vi "test-find-path.vi"() -> ()   [LabVIEW 2019]
uses:
  <vilib>/Rock Robotics/WPI/ThirdParty/JAS_Junk/TrajLib/TypeDef/TRANSLATION2D.ctl
  <vilib>/Rock Robotics/WPI/ThirdParty/MJansen/PathPlanner/TypeDef/PathPlannerGoalEndState.ctl
  <vilib>/Rock Robotics/WPI/ThirdParty/JAS_Junk/TrajLib/TypeDef/ROTATION2D.ctl
  <vilib>/Rock Robotics/WPI/ThirdParty/MJansen/PathPlanner/TypeDef/PathPlannerPath.ctl
  <vilib>/Rock Robotics/WPI/ThirdParty/MJansen/PathPlanner/TypeDef/PathPlannerRotationTarget.ctl
  <vilib>/Rock Robotics/WPI/ThirdParty/MJansen/PathPlanner/TypeDef/PathPlannerConstraintsZone.ctl
  <vilib>/Rock Robotics/WPI/ThirdParty/MJansen/PathPlanner/TypeDef/PathPlannerPathConstraints.ctl
  <vilib>/Rock Robotics/WPI/ThirdParty/MJansen/PathPlanner/TypeDef/PathPlannerEventMarker.ctl
  <vilib>/Rock Robotics/WPI/ThirdParty/MJansen/PathPlanner/TypeDef/PathPlannerCommandUtil.ctl
  <vilib>/Rock Robotics/WPI/ThirdParty/MJansen/PathPlanner/ENum/PathPlanner_CommandUtilType_ENUM.ctl
  <vilib>/Rock Robotics/WPI/ThirdParty/MJansen/PathPlanner/TypeDef/PathPlannerPathPoint.ctl
  <vilib>/Rock Robotics/WPI/ThirdParty/JAS_Junk/TrajLib/TypeDef/CHASSIS_SPEEDS.ctl
  <vilib>/Rock Robotics/WPI/ThirdParty/MJansen/PathPlanner/VI/PathPlanner_GridPosition_Get.vi
  <vilib>/Rock Robotics/WPI/ThirdParty/JAS_Junk/TrajLib/Translation2d_Create.vi
  <vilib>/Rock Robotics/WPI/ThirdParty/MJansen/PathPlanner/VI/PathPlanner_PathFinder_Globals.vi
  <vilib>/robotics/Navigation/shared/WorldMap/OccupancyGridWorldMap/NI_Robotics_OccupancyGridWorldMap.lvclass
  <vilib>/robotics/Navigation/shared/MapNode/AbstractDstarNode/NI_Robotics_AbstractDstarNode.lvclass
  <vilib>/Rock Robotics/WPI/ThirdParty/MJansen/PathPlanner/PathPlanner24.lvlib
  <vilib>/Rock Robotics/WPI/ThirdParty/JAS_Junk/TrajLib/Trajectory_Library.lvlib
panel:
  out "Extract Simplified Path Size":i32
  out "Do Reset Err Count":i64
  out "Do Minor Err Count":i64
  out "Do Major Err Count":i64
  out "Extract Path Size":i32
  out "Field":cluster{dbl[], dbl[]}[](graph)=[{array[568 elements], array[568 elements]}, {[1.65, 1.9499999999999997, 2.25, 2.55, 2.8499999999999996, 3.15, 3.4499999999999997, 3.7499999999999996, 4.05, 4.3500000000000005, 4.65, 4.95, 5.25, 5.55, 5.8500000000000005, 6.15, 6.45, 6.75, 7.05, 7.35, 7.65, 7.95, 8.25, 8.55, 8.85, 9.15, 9.45, 9.75, 10.05, 10.35, 10.65, 10.95, 11.25, 11.55, 11.85, 12.15, 12.45, 12.75, 13.05, 13.35, 13.65], [1.65, 1.65, 1.65, 1.65, 1.65, 1.65, 1.65, 1.65, 1.65, 1.65, 1.65, 1.65, 1.65, 1.65, 1.65, 1.65, 1.65, 1.65, 1.65, 1.65, 1.65, 1.65, 1.65, 1.65, 1.65, 1.65, 1.65, 1.65, 1.65, 1.65, 1.65, 1.65, 1.65, 1.65, 1.65, 1.65, 1.65, 1.65, 1.65, 1.65, 1.65]}, {[1.65, 13.65], [1.65, 1.65]}, {[1.5, 2.1072631250000002, 2.7161800000000005, 3.326566875, 3.9382400000000004, 4.551015625, 5.1647099999999995, 5.779139375, 6.39412, 7.009468125, 7.624999999999998, 8.240531874999999, 8.855879999999999, 9.470860625, 10.08529, 10.698984375000002, 11.311760000000003, 11.923433125000003, 12.533820000000002, 13.142736875000004, 13.75], [1.5, 1.5, 1.5, 1.5, 1.5, 1.5, 1.5, 1.5, 1.5, 1.5, 1.5, 1.5, 1.5, 1.5, 1.5, 1.5, 1.5, 1.5, 1.5, 1.5, 1.5]}, {array[568 elements], array[568 elements]}]
  out "Error_No_Path":bool
  out "New Path Available":bool
  out "Loop Count":i32
  out "TerminateWorker":bool
  out "Do Work Count":i64
  out "Do Reset Count":i64
  out "Do Minor Count":i64
  out "Do Major Count":i64
  out "PathPlannerPath":T1={"BezierPoints"=[], "PreviewStartingRotation"={"VALUE"=0.0, "COS"=1.0, "SIN"=0.0}, "Reversed"=FALSE, "RotationTargets"=[], "ConstraintZones"=[], "EventMarkers"=[], "GlobalConstraints"={"MaxVelocityMps;"=0.0, "MaxAccelerationMpsSq;"=0.0, "MaxAngularVelRadPsEc;"=0.0, "MaxAngularAccRadPSecSq"=0.0, "Exists"=FALSE}, "GoalEndState"={"Velocity"=0.0, "Rotation"={"VALUE"=0.0, "COS"=1.0, "SIN"=0.0}}, "AllPoints"=[]} {"AllPoints"."HolonomicRotation"."SIN" format="%13.4f"; "AllPoints"."HolonomicRotation"."COS" format="%13.4f"; "AllPoints"."HolonomicRotation"."VALUE" format="%13.4f"; "AllPoints"."Position"."Y" format="%14.3f"; "AllPoints"."Position"."X" format="%14.3f"; "GoalEndState"."Rotation"."SIN" format="%13.4f"; "GoalEndState"."Rotation"."COS" format="%13.4f"; "GoalEndState"."Rotation"."VALUE" format="%13.4f"; "EventMarkers"."lastRobotPos"."Y" format="%14.3f"; "EventMarkers"."lastRobotPos"."X" format="%14.3f"; "EventMarkers"."markerPos"."Y" format="%14.3f"; "EventMarkers"."markerPos"."X" format="%14.3f"; "RotationTargets"."target"."SIN" format="%13.4f"; "RotationTargets"."target"."COS" format="%13.4f"; "RotationTargets"."target"."VALUE" format="%13.4f"; "PreviewStartingRotation"."SIN" format="%13.4f"; "PreviewStartingRotation"."COS" format="%13.4f"; "PreviewStartingRotation"."VALUE" format="%13.4f"; "BezierPoints"."Y" format="%14.3f"; "BezierPoints"."X" format="%14.3f"}
  in  "GoalEndState":T10={"Velocity"=0.0, "Rotation"={"VALUE"=0.0, "COS"=1.0, "SIN"=0.0}} {"Rotation"."SIN" format="%13.4f"; "Rotation"."COS" format="%13.4f"; "Rotation"."VALUE" format="%13.4f"}
  in  "Goal Position":T2={"X"=14.0, "Y"=7.0} {"Y" step=0.25 format="%14.3f"; "X" step=0.25 format="%14.3f"}
  in  "StartPosition":T2={"X"=1.5, "Y"=1.5} {"Y" step=0.25 format="%14.3f"; "X" step=0.25 format="%14.3f"}
  out "NewPathAvailLastCheck":i32
  out "NewPathAvailCount":i32
  out "BackGroundInitialized":bool
  out "Main Program Name":string
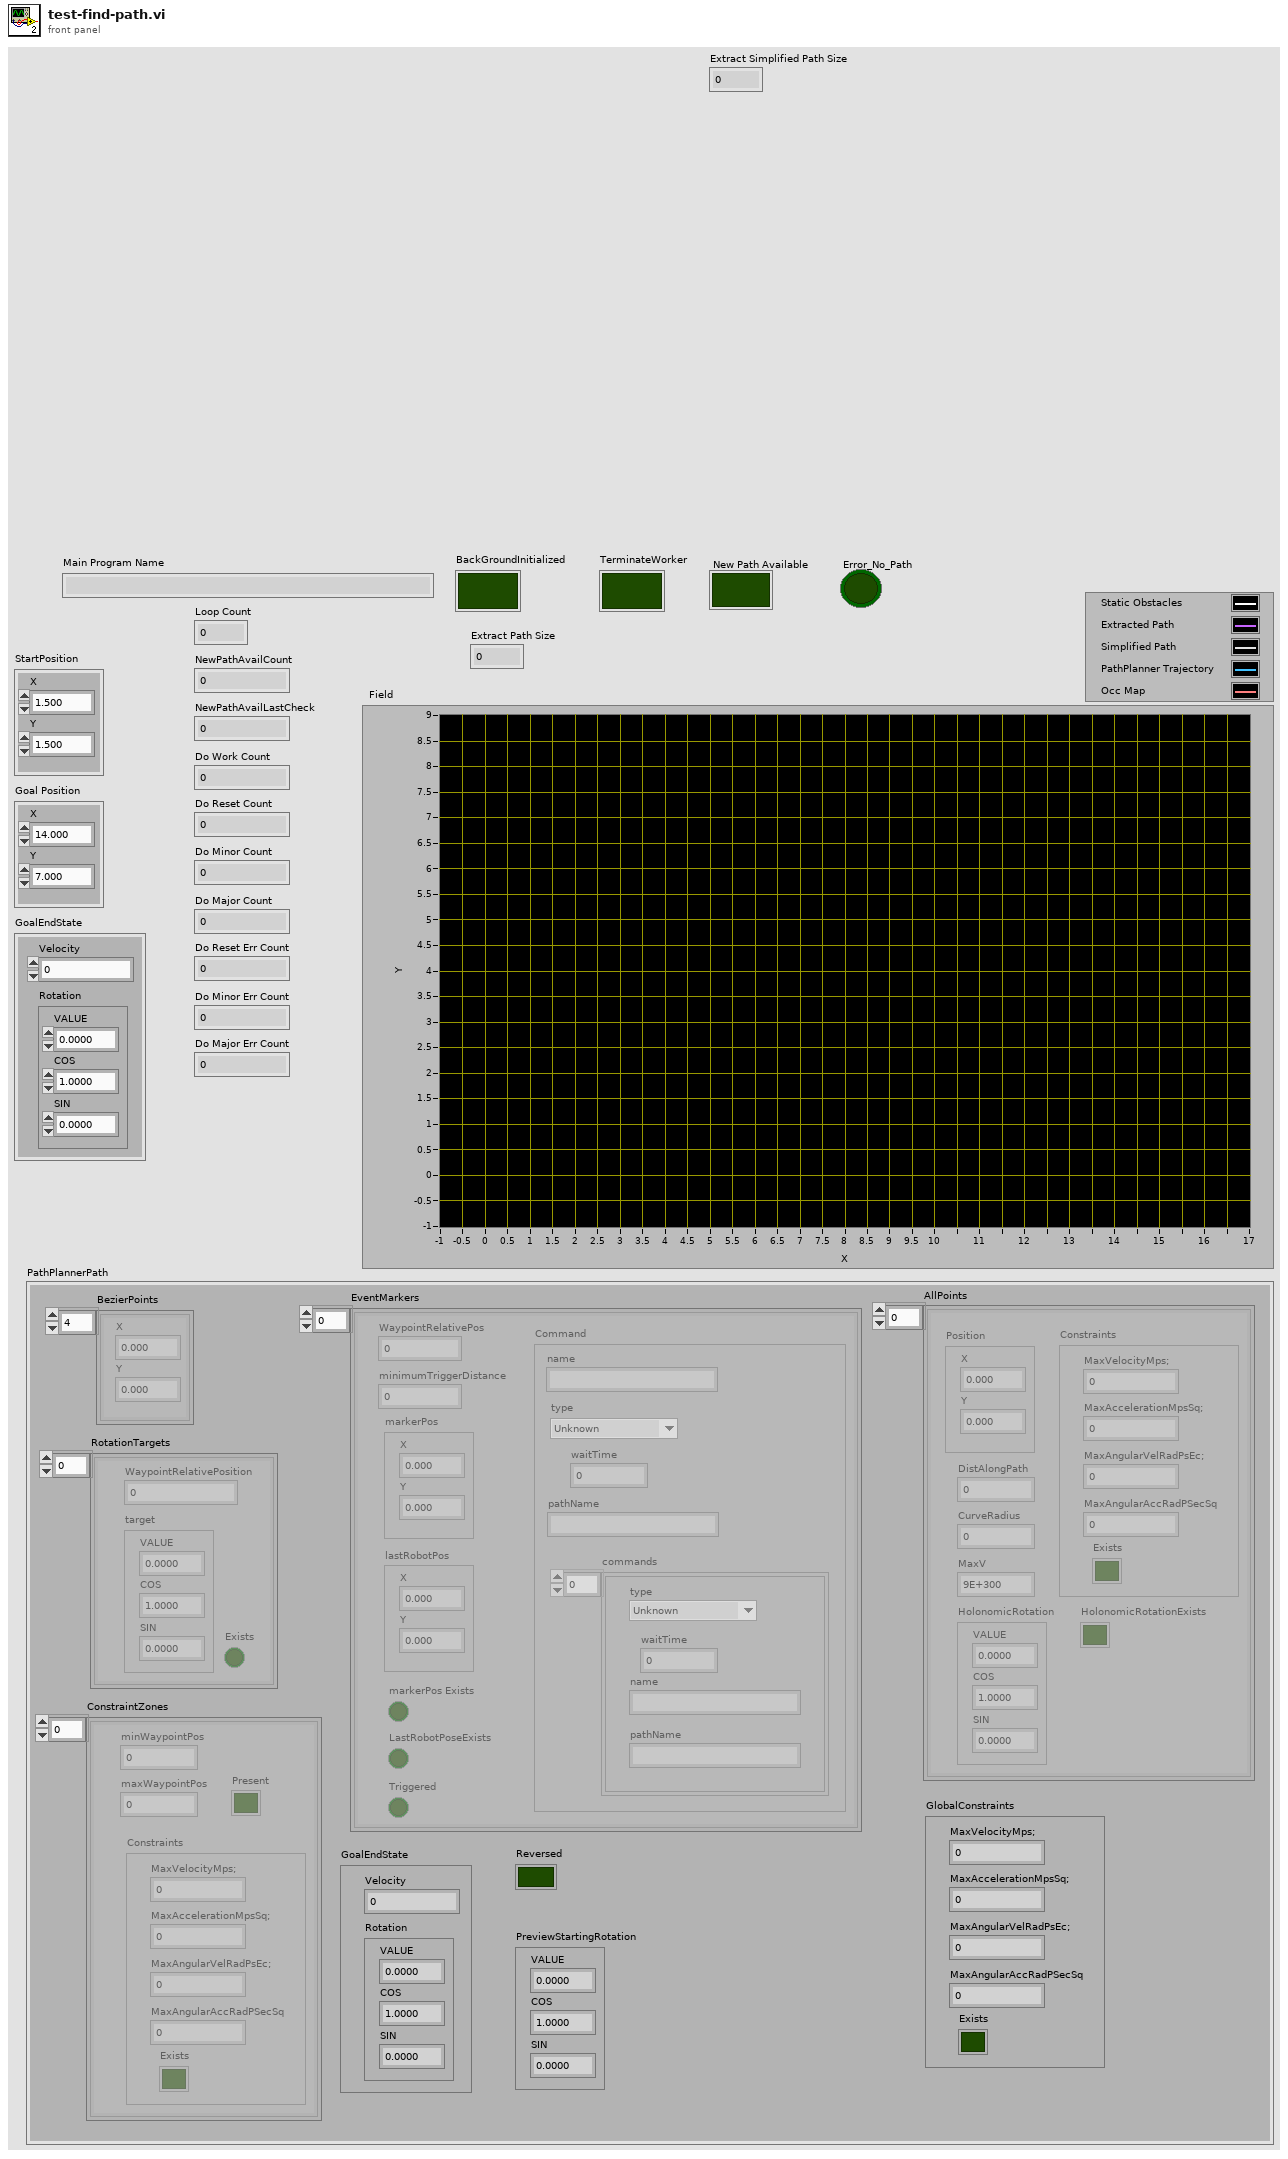
[diagram p1: front panel]
types:
  T1 = typedef "PathPlanner24.lvlib/PathPlannerPath.ctl" = cluster{"BezierPoints":T2[], "PreviewStartingRotation":T3, "Reversed":bool, "RotationTargets":T4[], "ConstraintZones":T5[], "EventMarkers":T7[], "GlobalConstraints":T6, "GoalEndState":T10, "AllPoints":T11[]}
  T2 = typedef "Trajectory_Library.lvlib/TRANSLATION2D.ctl" = cluster{"X":dbl, "Y":dbl}
  T3 = typedef "Trajectory_Library.lvlib/ROTATION2D.ctl" = cluster{"VALUE":dbl, "COS":dbl, "SIN":dbl}
  T4 = typedef "PathPlanner24.lvlib/PathPlannerRotationTarget.ctl" = cluster{"target":T3, "WaypointRelativePosition":dbl, "Exists":bool}
  T5 = typedef "PathPlanner24.lvlib/PathPlannerConstraintsZone.ctl" = cluster{"minWaypointPos":dbl, "maxWaypointPos":dbl, "Constraints":T6, "Present":bool}
  T6 = typedef "PathPlanner24.lvlib/PathPlannerPathConstraints.ctl" = cluster{"MaxVelocityMps;":dbl, "MaxAccelerationMpsSq;":dbl, "MaxAngularVelRadPsEc;":dbl, "MaxAngularAccRadPSecSq":dbl, "Exists":bool}
  T7 = typedef "PathPlanner24.lvlib/PathPlannerEventMarker.ctl" = cluster{"WaypointRelativePos":dbl, "minimumTriggerDistance":dbl, "markerPos":T2, "lastRobotPos":T2, "Command":T8, "markerPos Exists":bool, "LastRobotPoseExists":bool, "Triggered":bool}
  T8 = typedef "PathPlanner24.lvlib/PathPlannerCommandUtil.ctl" = cluster{"waitTime":dbl, "name":string, "pathName":string, "commands":cluster{"type":T9, "waitTime":dbl, "name":string, "pathName":string}[], "type":T9}
  T9 = typedef "PathPlanner24.lvlib/PathPlanner_CommandUtilType_ENUM.ctl" = enum16{"Unknown", "Wait", "Named", "Path", "Sequential", "Parallel", "Race", "Deadline"}
  T10 = typedef "PathPlanner24.lvlib/PathPlannerGoalEndState.ctl" = cluster{"Velocity":dbl, "Rotation":T3}
  T11 = typedef "PathPlanner24.lvlib/PathPlannerPathPoint.ctl" = cluster{"Position":T2, "HolonomicRotation":T3, "DistAlongPath":dbl, "CurveRadius":dbl, "MaxV":dbl, "Constraints":T6, "HolonomicRotationExists":bool}
  T12 = typedef "Trajectory_Library.lvlib/CHASSIS_SPEEDS.ctl" = cluster{"vX":dbl, "vY":dbl, "vOmega":dbl}
  T13 = cluster{"DoResetErrCount":i64, "DoResetCount":i64, "DoMinorErrCount":i64, "DoMinorCount":i64, "DoMajorErrCount":i64, "DoMajorCount":i64, "DoWorkLoopCount":i64, "BackGroundInitialized":bool, "TerminateWorker":bool}
  T14 = typedef "PathPlanner24.lvlib/PathPlannerFinderGridPosition.ctl" = cluster{"X":i32, "Y":i32}
  T15 = cluster{"ExtractedPath":T14[], "ExtractedPathSimplified":T14[], "ExtractedFieldPosPath":T2[], "CurrentPath":T2[], "Obstacles":set{T14}, "StaticOccupancyGrid":refnum<data-value>, "path references":refnum<data-value>[], "Main Program Name":string}
  T16 = typedef "PathPlanner24.lvlib/PathPlannerTrajectory.ctl" = cluster{"States":T17[]}
  T17 = typedef "PathPlanner24.lvlib/PathPlannerTrajectoryState.ctl" = cluster{"TimeSeconds":dbl, "VelocityMPS":dbl, "AccerationMpsSq":dbl, "HeadingAngularVelRadPerSec":dbl, "PositionMeters":T2, "Heading":T3, "TargetHolonomicRotation":T3, "CurvatureRadPerMeter":dbl, "PathPlannerConstraints":T6, "DeltaPos":dbl}
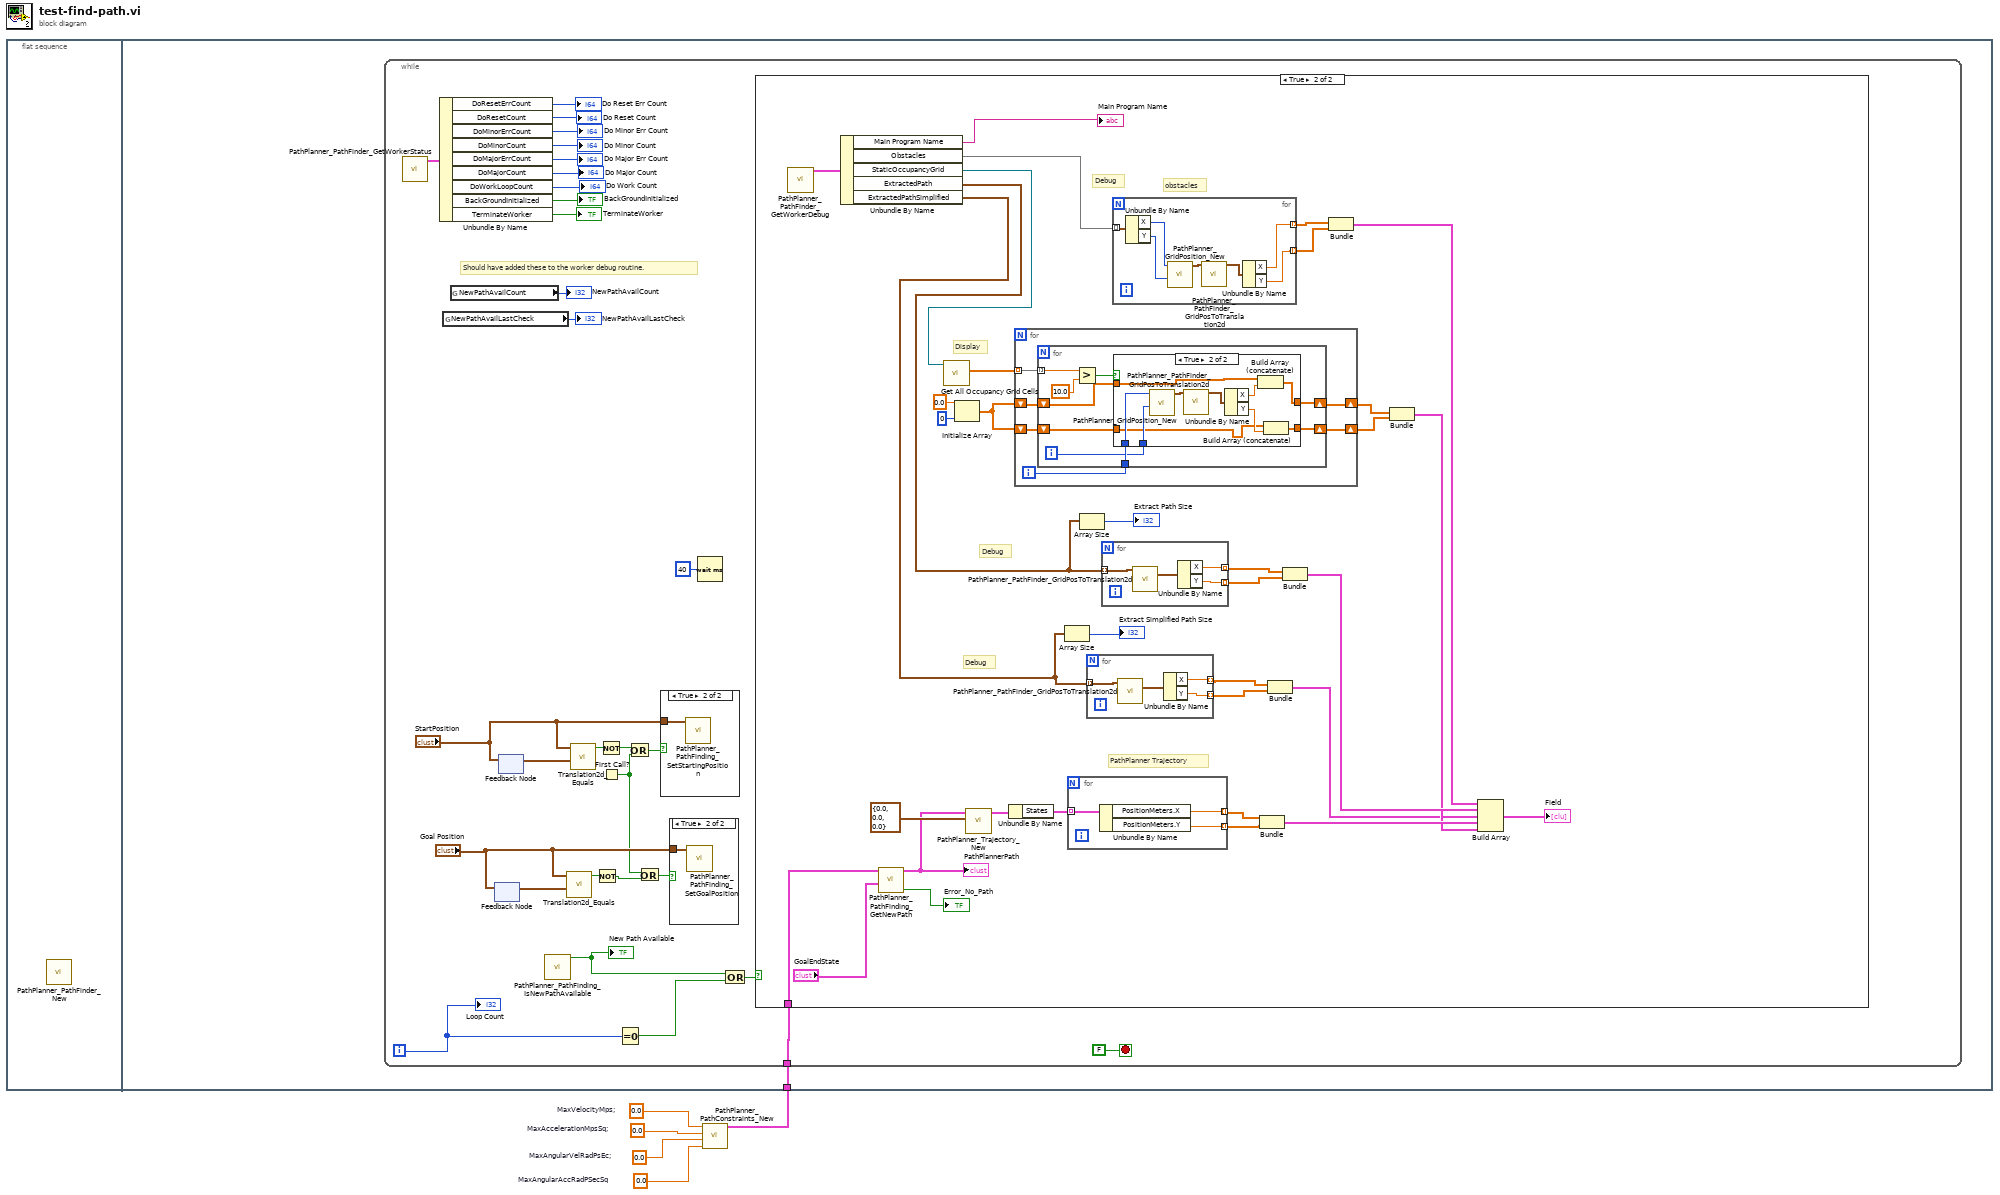
[diagram p0: block diagram]
diagram:
  w1 = 0.0  # MaxVelocityMps;
  w2 = 0.0  # MaxAccelerationMpsSq;
  w3 = 0.0  # MaxAngularVelRadPsEc;
  w4 = 0.0  # MaxAngularAccRadPSecSq
  n1 = flat-sequence {
    tunnel: w5 -> [w6]
    frame #0 {
      n2 = call <vilib>:"PathPlanner_PathFinder_New.vi"() -> ()  [unwired: 11 in, 1 out]
    }
    frame #1 {
      n3 = while {
        tunnel: w6 -> [w29]
        i -> [w31]
        stop <- FALSE stop-if-true
        # "Should have added these to the worker debug routine."
        n4 = call <vilib>:"PathPlanner_PathFinder_GetWorkerStatus.vi"() -> ("PathFindingWorkerStatus"=w16:T13)  [unwired: 11 in]
        n5 = Unbundle By Name(w16) -> ("DoResetErrCount"=→"Do Reset Err Count":i64, "DoResetCount"=→"Do Reset Count":i64, "DoMinorErrCount"=→"Do Minor Err Count":i64, "DoMinorCount"=→"Do Minor Count":i64, "DoMajorErrCount"=→"Do Major Err Count":i64, "DoMajorCount"=→"Do Major Count":i64, "DoWorkLoopCount"=→"Do Work Count":i64, "BackGroundInitialized"=→"BackGroundInitialized":bool, "TerminateWorker"=→"TerminateWorker":bool)
        n6 = global read "PathPlanner_PathFinder_Globals.vi" "NewPathAvailLastCheck"() -> (→"NewPathAvailLastCheck":i32)
        n7 = global read "PathPlanner_PathFinder_Globals.vi" "NewPathAvailCount"() -> (→"NewPathAvailCount":i32)
        n8 = feedback #1() -> (w33:T2)  [unwired: 1 in]
        n9 = feedback-in #1("Goal Position") -> ()
        n10 = feedback-in #2("StartPosition") -> ()
        n11 = feedback #2() -> (w35:T2)  [unwired: 1 in]
        n12 = call <vilib>:"PathPlanner_PathFinding_IsNewPathAvailable.vi"() -> ("New Path Available"=w26:bool)  [unwired: 11 in]
        "New Path Available" <- w26
        n13 = call <vilib>:"Translation2d_Equals.vi"("other Translation"=w33, "In Translation"="Goal Position") -> ("Equals"=w32:bool)  [unwired: 9 in]
        n14 = call <vilib>:"Translation2d_Equals.vi"("other Translation"=w35, "In Translation"="StartPosition") -> ("Equals"=w34:bool)  [unwired: 9 in]
        n15 = Not(x=w32) -> (.not. x?=w21:bool)
        n16 = Not(x=w34) -> (.not. x?=w19:bool)
        n17 = First Call?() -> (First Call?: T/F=w20:bool)
        n18 = Equal To 0?(x=w31) -> (x = 0?=w28:bool)
        n19 = Or(x=w19, y=w20) -> (x .or. y?=w23:bool)
        n20 = Or(x=w20, y=w21) -> (x .or. y?=w22:bool)
        n21 = case shown="True" w23 {
          tunnel: "StartPosition" -> [_ w118]
          frame False {
          }
          frame True {
            n22 = call <vilib>:"PathPlanner_PathFinding_SetStartingPosition.vi"("StartPosition"=w118) -> ()  [unwired: 11 in]
          }
        }
        n23 = case shown="True" w22 {
          tunnel: "Goal Position" -> [_ w117]
          frame False {
          }
          frame True {
            n24 = call <vilib>:"PathPlanner_PathFinding_SetGoalPosition.vi"("GoalPosition"=w117) -> ()  [unwired: 11 in]
          }
        }
        n25 = Wait (ms)(milliseconds to wait=u32 40) -> ()  [unwired: 1 out]
        n26 = Compound Arithmetic op=OR(w26, w28) -> (w30:bool)
        n27 = case shown="True" w30 {
          tunnel: w29 -> [_ w64]
          frame False {
          }
          frame True {
            # "Debug"
            # "Display"
            # "Debug"
            # "Debug"
            # "obstacles"
            # "PathPlanner Trajectory"
            n28 = call <vilib>:"PathPlanner_PathFinder_GetWorkerDebug.vi"() -> ("PathFinderWorkerDebug"=w42:T15)  [unwired: 11 in]
            n29 = Unbundle By Name(w42) -> ("Main Program Name"=→"Main Program Name":string, "Obstacles"=w40:set{T14}, "StaticOccupancyGrid"=w39:refnum<data-value>, "ExtractedPath"=w38:T14[], "ExtractedPathSimplified"=w37:T14[])
            n30 = call <vilib>:"PathPlanner_PathFinding_GetNewPath.vi"("GoalEndState"="GoalEndState", "PathPlannerPathConstraints"=w64) -> ("Error_No_Path"=→"Error_No_Path":bool, "PathPlannerPath"=w62:T1)  [unwired: 8 in]
            "PathPlannerPath" <- w62
            n31 = call <vilib>:"Get All Occupancy Grid Cells.vi"("map reference in"=w39) -> ("occupancy grid"=w46:dbl[][])  [unwired: 8 in, 2 out]
            n32 = Initialize Array(0.0 ("element"), 0 ("dimension size")) -> (w43:dbl[])
            n33 = call <vilib>:"PathPlanner_Trajectory_New.vi"("StartingSpeeds"=T12 {"vX"=0.0, "vY"=0.0, "vOmega"=0.0}, "Path"=w62) -> ("PathPlannerTrajectory"=w66:T16)  [unwired: 9 in]
            n34 = Unbundle By Name(w66) -> ("States"=w60:T17[])
            n35 = for {
              tunnel: w46 -> [w81] mode=indexing
              shift-right: [w77] -> w53
              shift-left: w43 -> [w80]
              shift-right: [w76] -> w52
              shift-left: w43 -> [w79]
              i -> [w78]
              n36 = for {
                tunnel: w81 -> [w90] mode=indexing
                shift-right: [w84] -> w77
                shift-left: w80 -> [w85]
                shift-right: [w82] -> w76
                shift-left: w79 -> [w83]
                tunnel: w78 -> [w87]
                i -> [w86]
                n37 = Greater?(x=w90, y=10.0) -> (0:w88:bool)
                n38 = case shown="True" w88 {
                  tunnel: w87 -> [_ w101]
                  tunnel: w86 -> [_ w97]
                  tunnel: w85 -> [w92 w96]
                  tunnel: [w92 w95] -> w84
                  tunnel: w83 -> [w91 w94]
                  tunnel: [w91 w93] -> w82
                  frame False {
                  }
                  frame True {
                    n39 = call <vilib>:"PathPlanner_GridPosition_New.vi"("Int Y"=w97, "Int X"=w101) -> ("GridPosition"=w102:T14)  [unwired: 9 in]
                    n40 = call <vilib>:"PathPlanner_PathFinder_GridPosToTranslation2d.vi"("GridPosition"=w102) -> ("RealGridPos"=w100:T2)  [unwired: 10 in]
                    n41 = Unbundle By Name(w100) -> ("X"=w99:dbl, "Y"=w98:dbl)
                    n42 = Build Array (concatenate)(w96, w99) -> (w95:dbl[])
                    n43 = Build Array (concatenate)(w94, w98) -> (w93:dbl[])
                  }
                }
              }
            }
            n44 = Array Size(array=w37) -> (size(s)=→"Extract Simplified Path Size":i32)
            n45 = for {
              tunnel: [w108] -> w57 mode=indexing
              tunnel: [w109] -> w56 mode=indexing
              tunnel: w60 -> [w107] mode=indexing
              n46 = Unbundle By Name(w107) -> ("PositionMeters.X"=w108:dbl, "PositionMeters.Y"=w109:dbl)
            }
            n47 = Array Size(array=w38) -> (size(s)=→"Extract Path Size":i32)
            n48 = for {
              tunnel: [w73] -> w50 mode=indexing
              tunnel: [w75] -> w49 mode=indexing
              tunnel: w37 -> [w72] mode=indexing
              n49 = call <vilib>:"PathPlanner_PathFinder_GridPosToTranslation2d.vi"("GridPosition"=w72) -> ("RealGridPos"=w74:T2)  [unwired: 10 in]
              n50 = Unbundle By Name(w74) -> ("X"=w73:dbl, "Y"=w75:dbl)
            }
            n51 = for {
              tunnel: [w104] -> w59 mode=indexing
              tunnel: [w106] -> w58 mode=indexing
              tunnel: w38 -> [w103] mode=indexing
              n52 = call <vilib>:"PathPlanner_PathFinder_GridPosToTranslation2d.vi"("GridPosition"=w103) -> ("RealGridPos"=w105:T2)  [unwired: 10 in]
              n53 = Unbundle By Name(w105) -> ("X"=w104:dbl, "Y"=w106:dbl)
            }
            n54 = for {
              tunnel: w40 -> [w116] mode=indexing
              tunnel: [w111] -> w70 mode=indexing
              tunnel: [w110] -> w71 mode=indexing
              n55 = Unbundle By Name(w116) -> ("X"=w113:i32, "Y"=w112:i32)
              n56 = call <vilib>:"PathPlanner_GridPosition_New.vi"("Int Y"=w112, "Int X"=w113) -> ("GridPosition"=w115:T14)  [unwired: 9 in]
              n57 = call <vilib>:"PathPlanner_PathFinder_GridPosToTranslation2d.vi"("GridPosition"=w115) -> ("RealGridPos"=w114:T2)  [unwired: 10 in]
              n58 = Unbundle By Name(w114) -> ("X"=w111:dbl, "Y"=w110:dbl)
            }
            n59 = Bundle(w57, w56) -> (w55:cluster{dbl[], dbl[]})  [unwired: 1 in]
            n60 = Bundle(w50, w49) -> (w47:cluster{dbl[], dbl[]})  [unwired: 1 in]
            n61 = Bundle(w59, w58) -> (w65:cluster{dbl[], dbl[]})  [unwired: 1 in]
            n62 = Bundle(w70, w71) -> (w68:cluster{dbl[], dbl[]})  [unwired: 1 in]
            n63 = Bundle(w53, w52) -> (w54:cluster{dbl[], dbl[]})  [unwired: 1 in]
            n64 = Build Array(w68, w65, w47, w55, w54) -> (→"Field":cluster{dbl[], dbl[]}[])
          }
        }
        "Loop Count" <- w31
      }
    }
  }
  n65 = call <vilib>:"PathPlanner_PathConstraints_New.vi"("MaxAngularAccRadPSecSq"=w4, "MaxAngularVelRadPsEc;"=w3, "MaxAccelerationMpsSq;"=w2, "MaxVelocityMps;"=w1) -> ("PathPlannerConstraints"=w5:T6)  [unwired: 7 in]
